vi "AnotherClass_Create.vi"(0 "reference in":refnum<class "AnotherClass.lvclass">, 5 "error in (no error)":errorcluster) -> (14 "reference out":refnum<class "AnotherClass.lvclass">, 19 "error out":errorcluster)   [LabVIEW 2017, in "AnotherClass.lvclass"]
uses:
  AnotherClass.lvclass
  C:/Program Files (x86)/National Instruments/LabVIEW 2017/vi.lib/addons/_AddQ/G#Object/G#Object.lvclass
  vi.lib/addons/_AddQ/G#Object/G#Object.lvclass
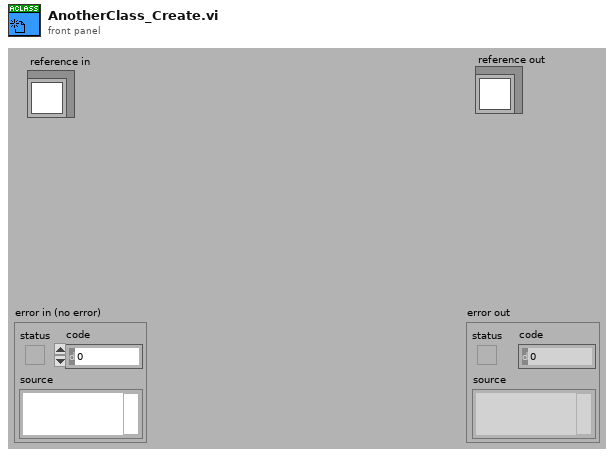
[diagram p1: front panel]
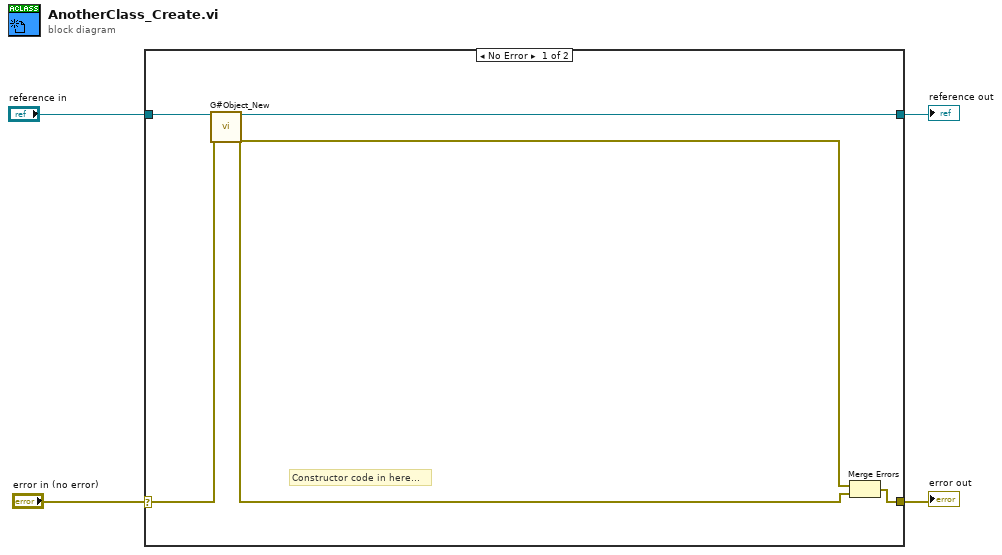
[diagram p0: block diagram]
diagram:
  n1 = case shown="No Error" "error in (no error)" {
    selector: "error in (no error)" -> [w9 w11]
    tunnel: [w7 w11] -> w4
    tunnel: "reference in" -> [w8 w10]
    tunnel: [w5 w10] -> w2
    frame No Error {
      # "Constructor code in here..."
      n2 = call "G#Object_New.vi"("reference in"=w8, "error in (no error)"=w9) -> ("reference out"=w5:refnum<class "AnotherClass.lvclass">, "error out"=w6:errorcluster)  [unwired: 15 in, 1 out]
      n3 = Merge Errors(w6, w6) -> (w7:errorcluster)
    }
    frame Error {
    }
  }
  "error out" <- w4
  "reference out" <- w2
